vi "Configure Frequency Sweep.vi"(0 "VISA resource name":refnum<visa-resource-name>, 1 "Enable Frequency Sweep (T: Enable)":bool=TRUE, 5 "Output Channel (1: Channel 1)":i32(ring)=1 items=["Channel 1"=1, "Channel 2"=2], 7 "Sweep Spacing (0: Linear)":i32(ring) items=["Linear", "Logarithmic", "Step"], 9 "Sweep Time (1 s)":dbl=1.0, 11 "error in (no error)":errorcluster, 12 "Start Frequency (100 Hz)":dbl=100.0, 13 "Stop Frequency (1000 Hz)":dbl=1000.0) -> (4 "VISA resource name out":refnum<visa-resource-name>, 15 "error out":errorcluster)   [LabVIEW 2012, in "RIGOL DG4000 Series.lvlib"]
doc: "Configures and enables a frequency sweep. In the frequency sweep mode, the function generator steps from the start frequency to the stop frequency at a sweep rate.\n\nNote:\nSweep mode must be enabled to perform a frequency sweep operation."
uses:
  <instrlib>/RIGOL DG4000 Series/RIGOL DG4000 Series.lvlib
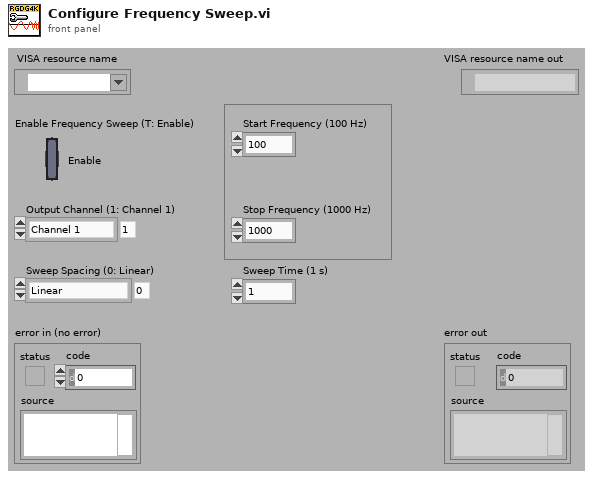
[diagram p1: front panel]
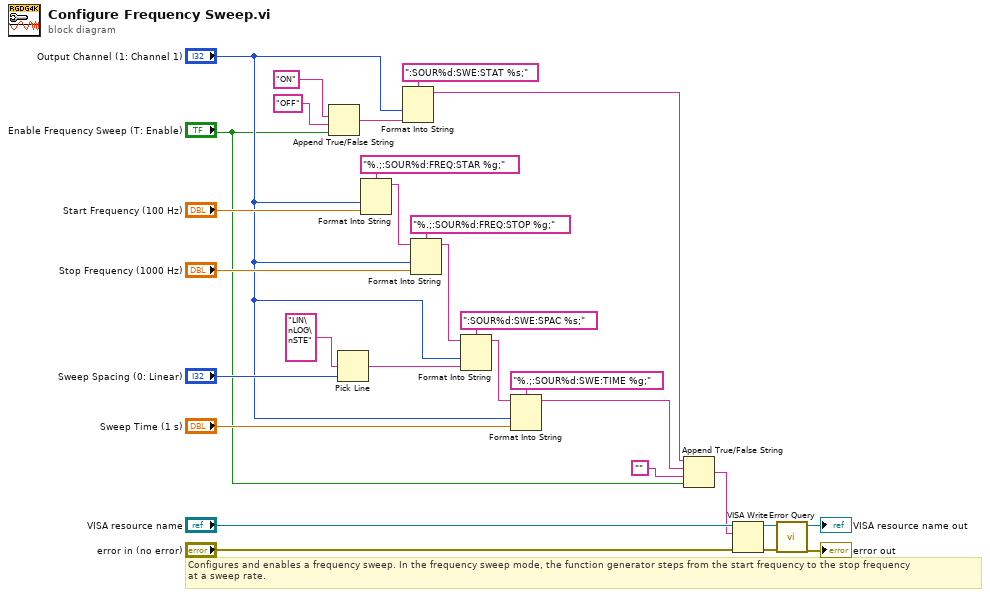
[diagram p0: block diagram]
diagram:
  # "Configures and enables a frequency sweep. In the frequency sweep mode, the function generator steps from the start frequency to the stop frequency \nat a sweep rate."
  n1 = Append True/False String(1:"Enable Frequency Sweep (T: Enable)", 2:"OFF", 3:"ON") -> (0:w13:string)  [unwired: 1 out]
  n2 = Pick Line(multi-line string="LIN\nLOG\nSTE", line index="Sweep Spacing (0: Linear)") -> (output string=w20:string)  [unwired: 1 out]
  n3 = Format Into String(format string="%.;:SOUR%d:FREQ:STAR %g;", "Output Channel (1: Channel 1)", "Start Frequency (100 Hz)") -> (resulting string=w27:string)  [unwired: 2 in, 1 out]
  n4 = Format Into String(format string=":SOUR%d:SWE:STAT %s;", "Output Channel (1: Channel 1)", w13) -> (resulting string=w4:string)  [unwired: 2 in, 1 out]
  n5 = Format Into String(format string="%.;:SOUR%d:FREQ:STOP %g;", initial string=w27, "Output Channel (1: Channel 1)", "Stop Frequency (1000 Hz)") -> (resulting string=w22:string)  [unwired: 1 in, 1 out]
  n6 = Format Into String(format string=":SOUR%d:SWE:SPAC %s;", initial string=w22, "Output Channel (1: Channel 1)", w20) -> (resulting string=w19:string)  [unwired: 1 in, 1 out]
  n7 = Format Into String(format string="%.;:SOUR%d:SWE:TIME %g;", initial string=w19, "Output Channel (1: Channel 1)", "Sweep Time (1 s)") -> (resulting string=w3:string)  [unwired: 1 in, 1 out]
  n8 = Append True/False String(1:"Enable Frequency Sweep (T: Enable)", 2:"", 3:w3, 4:w4) -> (0:w1:string)
  n9 = VISA Write(VISA resource name="VISA resource name", write buffer=w1, error in (no error)="error in (no error)") -> (VISA resource name out=w10:refnum<visa-resource-name>, error out=w9:errorcluster)  [unwired: 1 out]
  n10 = call <instrlib>:"Error Query.vi"("error in (no error)"=w9, "VISA resource name"=w10) -> ("error out"=→"error out":errorcluster, "VISA resource name out"=→"VISA resource name out":refnum<visa-resource-name>)  [unwired: 8 out]
